vi "Pipeline 4ch.vi"(8 "data in":T1[](array[typedef]), 9 "data in":T1[](array[typedef]), 10 "data in":T1[](array[typedef]), 11 "data in":T1[](array[typedef])) -> (0 "data out":T1[](array[typedef]), 1 "data out":T1[](array[typedef]), 2 "data out":T1[](array[typedef]), 3 "data out":T1[](array[typedef]))   [LabVIEW 2025, in "niUSRP Rx DSP v2 FPGA.lvclass"]
uses:
  niUSRP Rx DSP v2 FPGA.lvclass
  niUSRP Rx DSP v2 FPGA.lvclass/niUSRP Rx DSP v2 FPGA.ctl
  <instrlib>/_niInstr/DSP/v1/Shared/Public/IQ Data.ctl
  <instrlib>/_niInstr/DSP/v1/Shared/niInstr DSP v1 Shared.lvlib
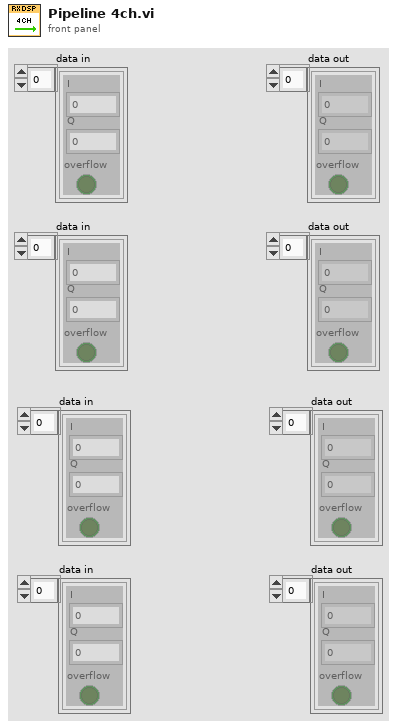
[diagram p1: front panel]
types:
  T1 = typedef "niInstr DSP v1 Shared.lvlib/IQ Data.ctl" = cluster{"I":fxp<+/-,18,1>, "Q":fxp<+/-,18,1>, "overflow":bool}
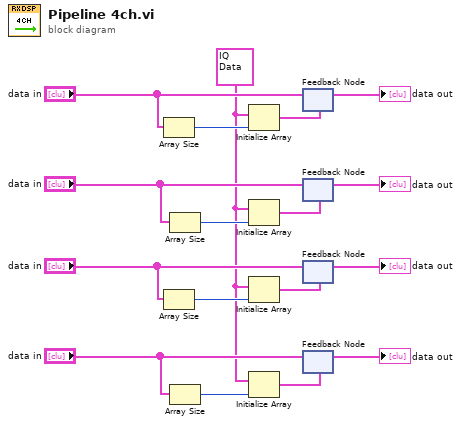
[diagram p0: block diagram]
diagram:
  w1 = T1 {"I"=0.0, "Q"=0.0, "overflow"=FALSE} ("data")
  n1 = Array Size(array="data in") -> (size(s)=w13:i32)
  n2 = Array Size(array="data in") -> (size(s)=w5:i32)
  n3 = Array Size(array="data in") -> (size(s)=w14:i32)
  n4 = Array Size(array="data in") -> (size(s)=w6:i32)
  n5 = Initialize Array(w1, w13) -> (w17:T1[])
  n6 = Initialize Array(w1, w14) -> (w16:T1[])
  n7 = Initialize Array(w1, w5) -> (w9:T1[])
  n8 = Initialize Array(w1, w6) -> (w8:T1[])
  n9 = feedback #1(w17) -> (→"data out":T1[])
  n10 = feedback-in #1("data in") -> ()
  n11 = feedback #2(w16) -> (→"data out":T1[])
  n12 = feedback-in #2("data in") -> ()
  n13 = feedback #3(w9) -> (→"data out":T1[])
  n14 = feedback-in #3("data in") -> ()
  n15 = feedback #4(w8) -> (→"data out":T1[])
  n16 = feedback-in #4("data in") -> ()
